vi "Logger_Message_Out.vi"(8 "error in (no error)":errorcluster caption="错误输入（无错误）", 10 "LoggerQueueRef":refnum<queue>, 11 "Logger 输入":refnum<class "Logger.lvclass">) -> (0 "error out":errorcluster caption="错误输出", 2 "Message":T1, 3 "Logger 输出":refnum<class "Logger.lvclass">)   [LabVIEW 2019, in "Logger.lvclass"]
uses:
  <userlib>/Logger/Logger.lvclass
  <userlib>/Logger/Ctls/LoggerMessage.ctl
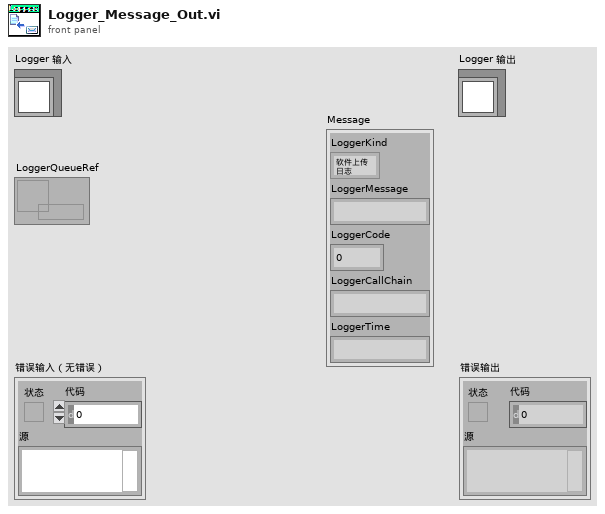
[diagram p1: front panel]
types:
  T1 = typedef "Logger.lvclass/LoggerMessage.ctl" = cluster{"LoggerKind":enum16{"软件上传日志", "软件其他日志", "软件错误日志", "软件监控日志"}, "LoggerMessage":string, "LoggerCode":i32, "LoggerCallChain":string, "LoggerTime":string}
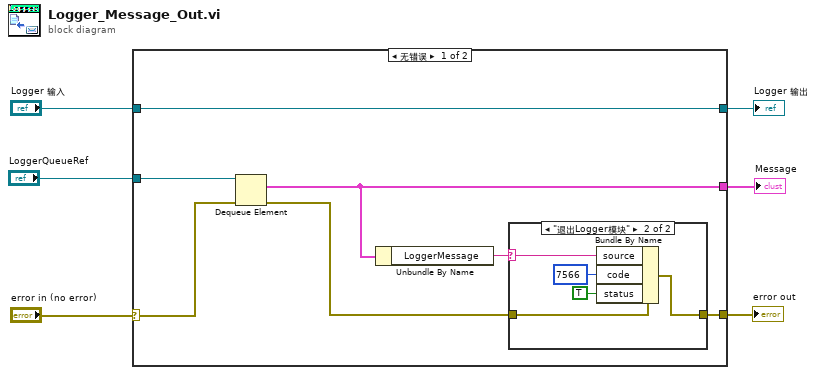
[diagram p0: block diagram]
diagram:
  n1 = case shown="无错误" "error in (no error)" {
    selector: "error in (no error)" -> [w11 w21]
    tunnel: [w7 w21] -> w5
    tunnel: [w13 w20] -> w3
    tunnel: "Logger 输入" -> [w13 w20]
    tunnel: "LoggerQueueRef" -> [w12 _]
    tunnel: [w9 _] -> w1
    frame No Error {
      n2 = Dequeue Element(queue=w12, error in (no error)=w11) -> (element=w9:T1, error out=w8:errorcluster)  [unwired: 1 in, 2 out]
      n3 = Unbundle By Name(w9) -> ("LoggerMessage"=w10:string)
      n4 = case shown="\"退出Logger模块\"" w10 {
        selector: w10 -> [_ w18]
        tunnel: w8 -> [w14 w19]
        tunnel: [w14 w17] -> w7
        frame "message", Default {
        }
        frame "退出Logger模块" {
          n5 = Bundle By Name(cluster=w19, "source"=w18, "code"=7566, "status"=TRUE) -> (w17:errorcluster)
        }
      }
    }
    frame Error {
    }
  }
  "error out" <- w5
  "Logger 输出" <- w3
  "Message" <- w1
